vi "QWTB Algorithms Filter Find Existing Algs.vi"(10 "exclude algs list":string[](array[string]), 11 "QWTB path":path) -> (3 "available algs list":string[](array[string]))   [LabVIEW 2020]
uses:
  6119a057-72d7-40d8-9562-c1e8ed5ed6b9.vi
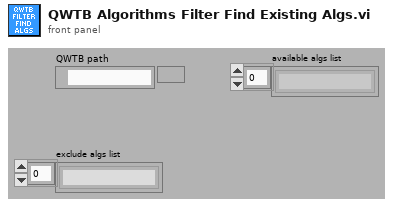
[diagram p1: front panel]
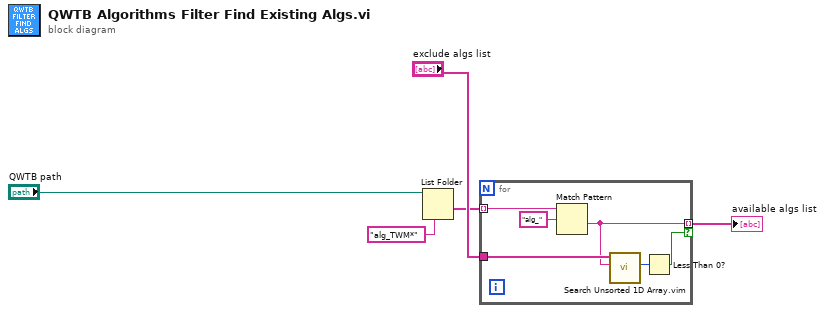
[diagram p0: block diagram]
diagram:
  n1 = List Folder(path="QWTB path", pattern="alg_TWM*") -> (folder names=w3:string[])  [unwired: 2 in, 3 out]
  n2 = for {
    tunnel: w3 -> [w11] mode=indexing
    tunnel: [w8] -> w4 mode=indexing if=w6
    tunnel: "exclude algs list" -> [w9]
    n3 = Match Pattern(string=w11, regular expression="alg_") -> (after substring=w8:string)  [unwired: 1 in, 3 out]
    n4 = call "Search Unsorted 1D Array.vim"("element"=w8, "unsorted 1D array"=w9) -> ("index of element"=w7:i32)  [unwired: 9 in]
    n5 = Less Than 0?(x=w7) -> (x < 0?=w6:bool)
  }
  "available algs list" <- w4
